vi "Get Path Loss.vi"(4 "Calibration Enabled":bool, 6 "Frequency":dbl, 7 "Data File Format":string="TwoColumnText", 8 "error in (no error)":errorcluster, 9 "Power Level":dbl, 11 "Normalization Files":path[](array[path])) -> (0 "error out":errorcluster, 1 "Adjusted Power Level":dbl, 2 "Correction Factor (dB)":dbl, 3 "Cal Data Folder":path, 5 "Route Names":string[](array[string]))   [LabVIEW 2015]
doc: "This VI will search the Cal data folder for calibration data file with the route name, it will then extract the route path loss at interpolated at the frequency of interest. Data will be maintained in memory, file is read in only once.\nRoute Name must be a valid route name from Switch Executive configuration."
uses:
  <vilib>/Utility/file.llb/Read From Spreadsheet File (DBL).vi
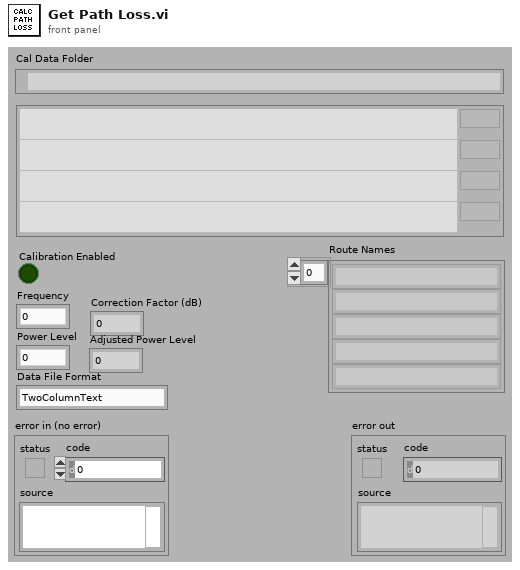
[diagram p1: front panel]
types:
  T1 = cluster{string, "all rows":dbl[], "all rows":dbl[]}
  T2 = cluster{string, "all rows":dbl[], "all rows":dbl[]}[]
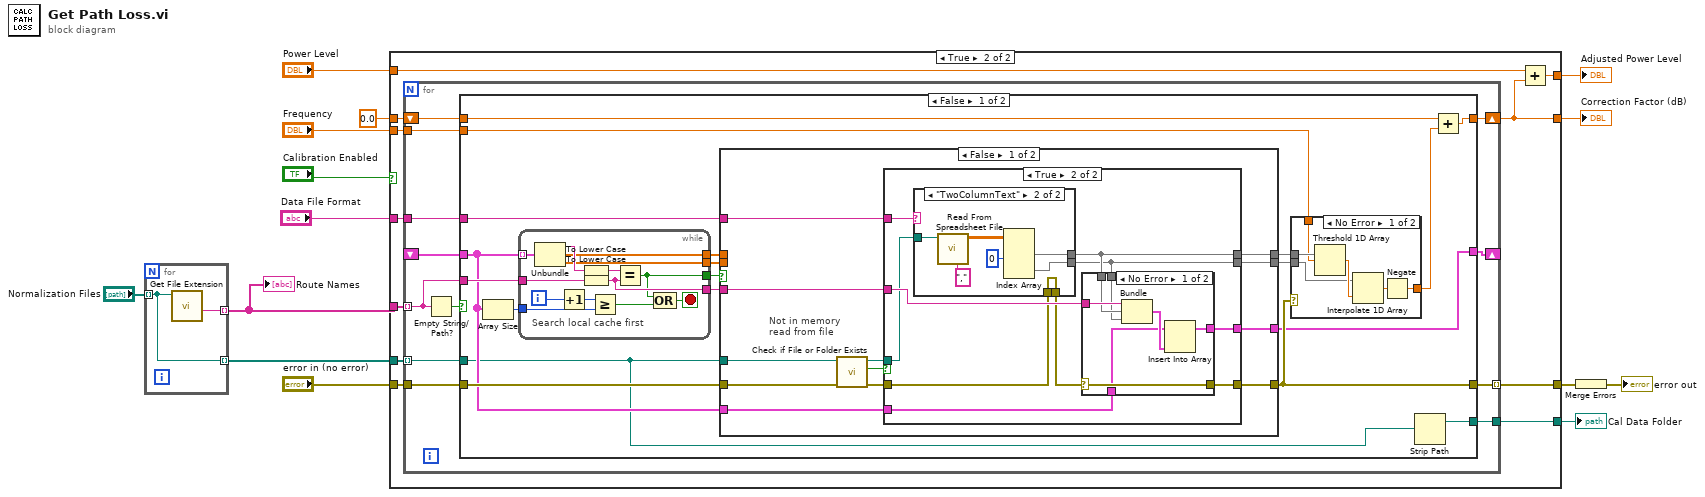
[diagram p0: block diagram]
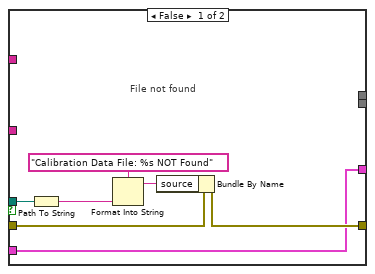
[diagram p4: hidden frame]
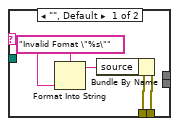
[diagram p6: hidden frame]
diagram:
  n1 = for {
    tunnel: "Normalization Files" -> [w15] mode=indexing
    tunnel: [w16] -> w2 mode=indexing
    tunnel: [w15] -> w1 mode=indexing
    n2 = call <vilib>:"Get File Extension.vi"("file"=w15) -> ("filename without extension"=w16:string)  [unwired: 6 in, 4 out]
  }
  "Route Names" <- w2
  n3 = case shown="True" "Calibration Enabled" {
    tunnel: 0.0 -> [w17 w29]
    tunnel: "error in (no error)" -> [_ w28]
    tunnel: [w17 w20] -> w13
    tunnel: [_ w27] -> w12
    tunnel: "Frequency" -> [_ w26]
    tunnel: "Data File Format" -> [_ w25]
    tunnel: w2 -> [_ w24]
    tunnel: [_ w23] -> w8
    tunnel: "Power Level" -> [w18 w22]
    tunnel: [w18 w21] -> w4
    tunnel: w1 -> [_ w19]
    frame False {
    }
    frame True {
      n4 = for {
        tunnel: [w39] -> w23 mode=indexing
        tunnel: w28 -> [w38]
        tunnel: [w37] -> w27
        tunnel: w26 -> [w36]
        tunnel: w25 -> [w35]
        tunnel: w24 -> [w31] mode=indexing
        shift-right: [w40] -> w20
        shift-left: w29 -> [w41]
        shift-right: [w32] -> _
        shift-left: _ -> [w33]
        tunnel: w19 -> [w30] mode=indexing
        n5 = Empty String/Path?(string/path=w31) -> (empty?=w34:bool)
        n6 = case shown="False" w34 {
          tunnel: w41 -> [w53 w136]
          tunnel: [w52 w136] -> w40
          tunnel: [w48 w135] -> w39
          tunnel: w38 -> [w46 w135]
          tunnel: [w42 _] -> w37
          tunnel: w36 -> [w51 _]
          tunnel: w35 -> [w50 _]
          tunnel: w31 -> [w47 _]
          tunnel: w33 -> [w44 w134]
          tunnel: [w45 w134] -> w32
          tunnel: w30 -> [w43 _]
          frame False {
            n7 = Array Size(array=w44) -> (size(s)=w60:i32)
            n8 = while {
              tunnel: w44 -> [w133] mode=indexing
              tunnel: w47 -> [w132]
              tunnel: w60 -> [w128]
              tunnel: [w122] -> w58
              tunnel: [w121] -> w57
              tunnel: [w124] -> w59
              tunnel: [w127] -> w54
              i -> [w130]
              stop <- w125 stop-if-true
              # "Search local cache first"
              n9 = Unbundle(w133) -> (w123:string, "all rows"=w122:dbl[], "all rows"=w121:dbl[])
              n10 = Increment(x=w130) -> (x+1=w129:i32)
              n11 = To Lower Case(string=w123) -> (all lower case string=w131:string)
              n12 = To Lower Case(string=w132) -> (all lower case string=w127:string)
              n13 = Greater Or Equal?(x=w129, y=w128) -> (x >= y?=w126:bool)
              n14 = Equal?(x=w131, y=w127) -> (x = y?=w124:bool)
              n15 = Compound Arithmetic op=OR(w124, w126) -> (w125:bool)
            }
            n16 = case shown="False" w59 {
              tunnel: w58 -> [_ w120]
              tunnel: w57 -> [_ w119]
              tunnel: [w78 w120] -> w56
              tunnel: [w77 w119] -> w55
              tunnel: w54 -> [w68 _]
              tunnel: [w75 w118] -> w48
              tunnel: w50 -> [w74 _]
              tunnel: w46 -> [w71 w118]
              tunnel: [w72 w117] -> w45
              tunnel: w44 -> [w69 w117]
              tunnel: w43 -> [w67 _]
              frame False {
                # "Not in memory\nread from file"
                n17 = call <vilib>:"Check if File or Folder Exists.vi"("error in (no error)"=w71, "path"=w67) -> ("error out"=w70:errorcluster, "file or folder exists?"=w76:bool, "dup path"=w73:path)  [unwired: 7 in]
                n18 = case shown="True" w76 {
                  tunnel: w68 -> [_ w95]
                  tunnel: [_ w94] -> w78
                  tunnel: [_ w93] -> w77
                  tunnel: w73 -> [w84 w92]
                  tunnel: [w81 w90] -> w75
                  tunnel: w74 -> [_ w91]
                  tunnel: [w80 w89] -> w72
                  tunnel: w70 -> [w79 w87]
                  tunnel: w69 -> [w80 w86]
                  frame False {
                    # "File not found"
                    n19 = Path To String(path=w84) -> (string=w83:string)
                    n20 = Format Into String(format string="Calibration Data File: %s NOT Found", w83) -> (resulting string=w82:string)  [unwired: 2 in, 1 out]
                    n21 = Bundle By Name(cluster=w79, "source"=w82) -> (w81:errorcluster)
                  }
                  frame True {
                    n22 = case shown="\"TwoColumnText\"" w91 {
                      selector: w91 -> [w108 _]
                      tunnel: [_ w114] -> w94
                      tunnel: [_ w113] -> w93
                      tunnel: w92 -> [_ w112]
                      tunnel: [w106 w110] -> w88
                      tunnel: w87 -> [w105 w110]
                      frame "", Default {
                        n23 = Format Into String(format string="Invalid Fomat \"%s\"" ("source"), w108) -> (resulting string=w107:string)  [unwired: 2 in, 1 out]
                        n24 = Bundle By Name(cluster=w105, "source"=w107) -> (w106:errorcluster)
                      }
                      frame "TwoColumnText" {
                        n25 = call-poly <vilib>:"Read From Spreadsheet File.vi"("delimiter (\\t)"="," ("delimiter (\\t)"), "file path (dialog if empty)"=w112) -> ("all rows"=w116:dbl[][])  [unwired: 5 in, 4 out]
                        n26 = Index Array(array=w116, index (col) #1=0 ("disabled index (col)")) -> (element #1=w114:dbl[], element #2=w113:dbl[])  [unwired: 3 in]
                      }
                    }
                    n27 = case shown="No Error" w88 {
                      selector: w88 -> [w98 w104]
                      tunnel: w95 -> [w102 _]
                      tunnel: w94 -> [w101 _]
                      tunnel: w93 -> [w100 _]
                      tunnel: [w98 w104] -> w90
                      tunnel: [w97 w103] -> w89
                      tunnel: w86 -> [w96 w103]
                      frame No Error {
                        n28 = Bundle(w102, "all rows"=w101, "all rows"=w100) -> (w99:T1)  [unwired: 1 in]
                        n29 = Insert Into Array(array=w96, new element=w99) -> (w97:T2)  [unwired: 1 in]
                      }
                      frame Error {
                      }
                    }
                  }
                }
              }
              frame True {
                # "Found in memory"
              }
            }
            n30 = case shown="No Error" w48 {
              tunnel: w56 -> [w65 _]
              tunnel: w55 -> [w64 _]
              tunnel: w51 -> [w61 _]
              tunnel: [w62 _] -> w49
              frame No Error {
                n31 = Threshold 1D Array(2:w61, 3:w65) -> (0:w66:dbl)  [unwired: 1 in]
                n32 = Interpolate 1D Array(1:w66, 2:w64) -> (0:w63:dbl)
                n33 = Negate(x=w63) -> (-x=w62:dbl)
              }
              frame Error {
              }
            }
            n34 = Strip Path(path=w43) -> (stripped path=w42:path)  [unwired: 1 out]
            n35 = Add(x=w53, y=w49) -> (x+y=w52:dbl)
          }
          frame True, Default {
          }
        }
      }
      n36 = Add(x=w22, y=w20) -> (x+y=w21:dbl)
    }
  }
  "Adjusted Power Level" <- w4
  "Correction Factor (dB)" <- w13
  "Cal Data Folder" <- w12
  n37 = Merge Errors(w8) -> (→"error out":errorcluster)
